vi "UnexpectedDepsCheck.vi"(8 "error in (no error)":errorcluster) -> (0 "error out":errorcluster)   [LabVIEW 2023, in "CICD.lvlib"]
uses:
  CICD.lvlib
panel:
  in  "Library Name":string="ModuleA"
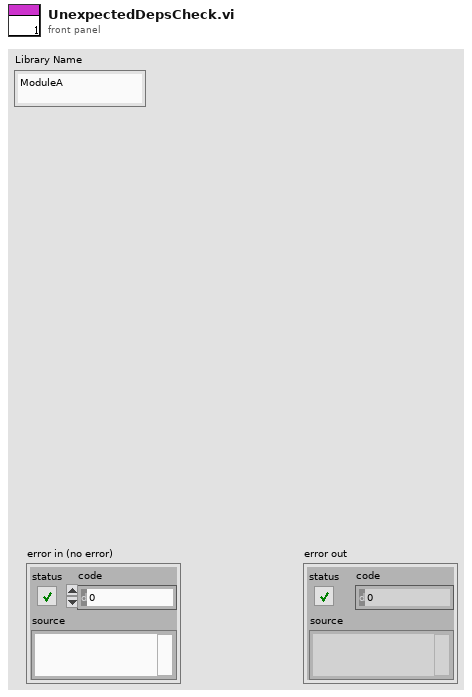
[diagram p1: front panel]
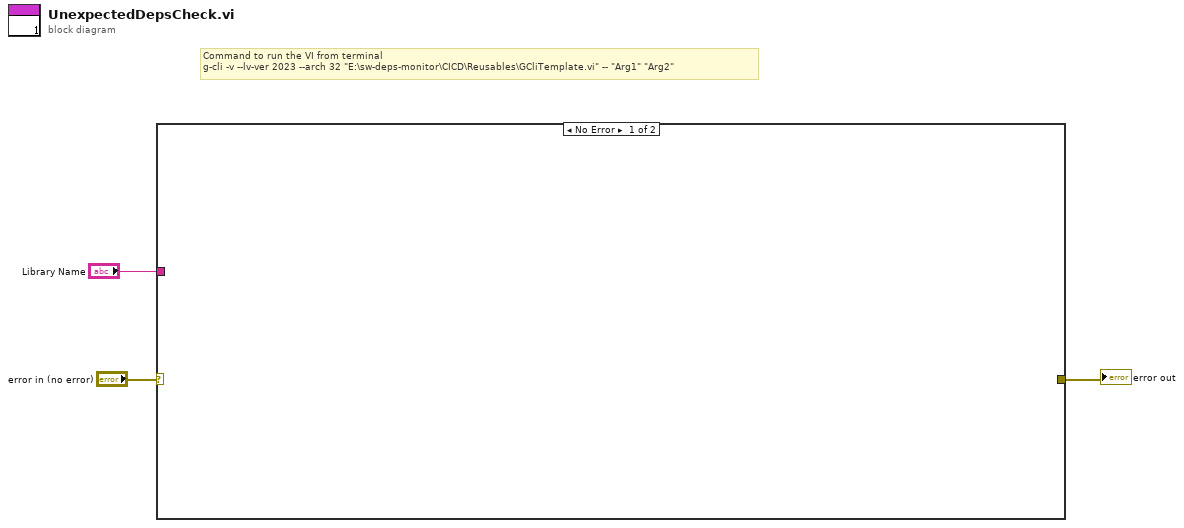
[diagram p0: block diagram]
diagram:
  # "Command to run the VI from terminal\ng-cli -v --lv-ver 2023 --arch 32 \"E:\\sw-deps-monitor\\CICD\\Reusables\\GCliTemplate.vi\" -- \"Arg1\" \"Arg2\""
  n1 = case shown="No Error" "error in (no error)" {
    selector: "error in (no error)" -> [_ w4]
    tunnel: [_ w4] -> w2
    tunnel: "Library Name" -> [_ _]
    frame No Error {
    }
    frame Error {
    }
  }
  "error out" <- w2
